vi "Get PGSQL datatype.vi"(8 "error in (no error)":errorcluster, 9 "Column Name":string, 10 "Table Path":string, 11 "LV-Data.PGSQL in":refnum<class "LV-Data.PGSQL.lvclass">) -> (0 "error out":errorcluster, 2 "Datatype":string, 3 "LV-Data.PGSQL out":refnum<class "LV-Data.PGSQL.lvclass">)   [LabVIEW 2016, in "LV-Data.PGSQL.lvclass"]
uses:
  LV-Data.PGSQL.lvclass
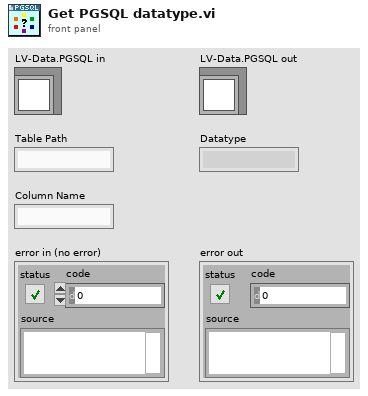
[diagram p1: front panel]
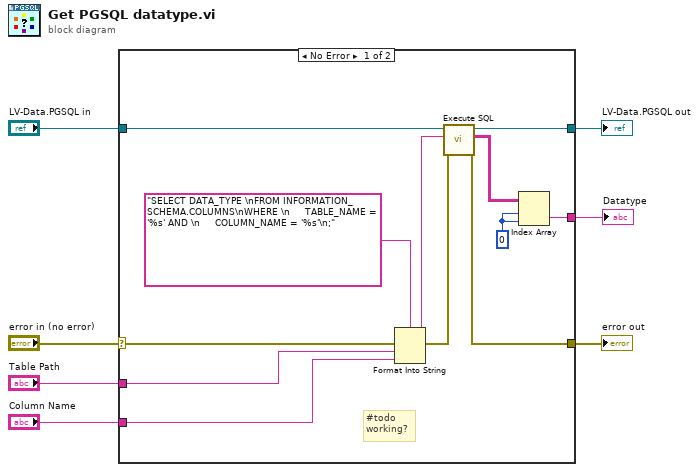
[diagram p0: block diagram]
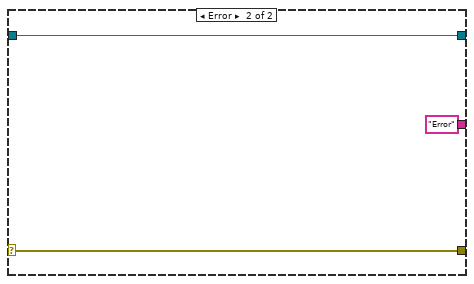
[diagram p2: hidden frame]
diagram:
  n1 = case shown="No Error" "error in (no error)" {
    selector: "error in (no error)" -> [w13 w22]
    tunnel: "Column Name" -> [w14 _]
    tunnel: [w11 w22] -> w7
    tunnel: [w12 w20] -> w5
    tunnel: "Table Path" -> [w15 _]
    tunnel: [w10 "Error" ("Get:Get String")] -> w2
    tunnel: "LV-Data.PGSQL in" -> [w9 w20]
    frame No Error {
      w17 = 0 ("index (row)")
      # "#todo\nworking?"
      n2 = Format Into String(format string="SELECT DATA_TYPE \nFROM INFORMATION_SCHEMA.COLUMNS\nWHERE \n     TABLE_NAME = '%s' AND \n     COLUMN_NAME = '%s'\n;", error in=w13, w15, w14) -> (resulting string=w8:string, error out=w16:errorcluster)  [unwired: 1 in]
      n3 = call "Execute SQL.vi"("error in"=w16, "SQL"=w8, "LV-Data.PGSQL"=w9) -> ("error out"=w11:errorcluster, "Result"=w19:string[][], "LV-Data.PGSQL out"=w12:refnum<class "LV-Data.PGSQL.lvclass">)  [unwired: 6 in]
      n4 = Index Array(array=w19, index (row)=w17, index (col)=w17) -> (element=w10:string)
    }
    frame Error {
    }
  }
  "error out" <- w7
  "LV-Data.PGSQL out" <- w5
  "Datatype" <- w2
